vi "GE5565 Enable DMA Interrupt (Cluster) Multi.vi"(4 "error in (no error)":errorcluster, 6 "transfer size (1024 bytes)":u32=1024, 7 "VMIC reference in":T1) -> (0 "error out":errorcluster, 3 "VMIC reference out":T1)   [LabVIEW 2020, in "RefMem DMA Engine.lvlib"]
uses:
  RefMem DMA Engine.lvlib
  <vilib>/Instr/_visa.llb/Select Event Type.ctl
  <vilib>/Instr/_visa.llb/VISA Register Access Address Space.ctl
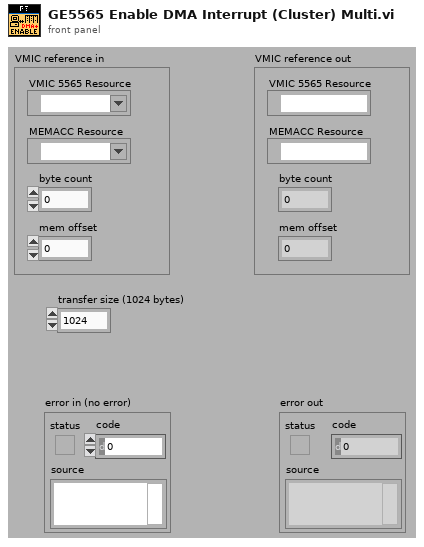
[diagram p1: front panel]
types:
  T1 = cluster{"VMIC 5565 Resource":refnum<visa-resource-name>, "MEMACC Resource":refnum<visa-resource-name>, "byte count":u32, "mem offset":u32}
  T2 = typedef "Select Event Type.ctl" = u32
  T3 = typedef "VISA Register Access Address Space.ctl" = u16
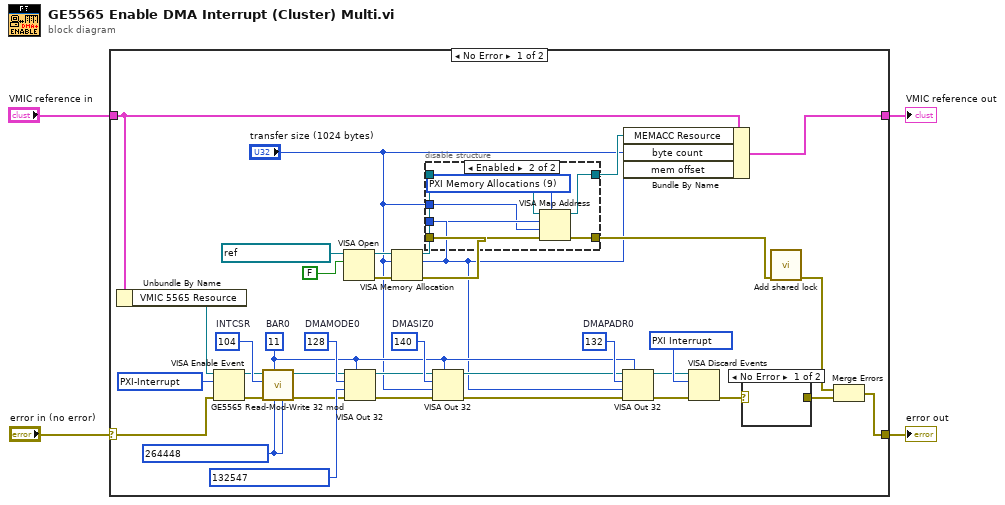
[diagram p0: block diagram]
diagram:
  n1 = case shown="No Error" "error in (no error)" {
    selector: "error in (no error)" -> [w27 w52]
    tunnel: "VMIC reference in" -> [w18 w53]
    tunnel: [w17 w53] -> w1
    tunnel: [w29 w52] -> w3
    frame No Error {
      w25 = u16 11  # BAR0
      w16 = T2 1073684514 items=["Service Request"=1073684491, "Trigger"=3221168138, "Clear"=1073684493, "VXI Signal"=1073684512, "VXI/VME Interrupt"=3221168161, "VXI/VME Sysfail"=1073684509, "VXI/VME Sysreset"=1073684510, "GPIB CIC"=1073684498, "GPIB Talk"=1073684499, "GPIB Listen"=1073684500, "PXI Interrupt"=1073684514, "Serial Break"=1073684515, "Serial TermChar"=1073684516, "Serial CTS"=1073684521, "Serial DSR"=1073684522, "Serial DCD"=1073684524, "Serial RI"=1073684526, "Serial Character"=1073684533, "USB Interrupt"=1073684535, "All Enabled"=1073709055] ("Event Type")
      w26 = u32 104  # INTCSR
      w24 = u32 264448 ("value")
      w28 = T2 1073684514 items=["ServiceRequest"=1073684491, "Trigger"=3221168138, "Clear"=1073684493, "VXI-Signal"=1073684512, "VXI/VME-Interrupt"=3221168161, "VXI/VME-Sysfail"=1073684509, "VXI/VME-Sysreset"=1073684510, "GPIB-CIC"=1073684498, "GPIB-Talk"=1073684499, "GPIB-Listen"=1073684500, "PXI-Interrupt"=1073684514, "AllEnabled"=1073709055] ("Event Type")
      w32 = u32 132  # DMAPADR0
      w35 = u32 140  # DMASIZ0
      w37 = u32 128  # DMAMODE0
      n2 = Unbundle By Name(w18) -> ("VMIC 5565 Resource"=w19:refnum<visa-resource-name>)
      n3 = VISA Enable Event(8:w27, 10:w28, 11:w19) -> (0:w23:errorcluster, 3:w22:refnum<visa-resource-name>)  [unwired: 1 in]
      n4 = call "GE5565 Read-Mod-Write 32 mod.vi"("value"=w24, "inv bit mask"=w24, "address space (13: BAR2)"=w25, "error in (no error)"=w23, "offset (0)"=w26, "VISA resource name"=w22) -> ("error out"=w20:errorcluster, "VISA resource name out"=w21:refnum<visa-resource-name>)  [unwired: 4 in]
      n5 = VISA Open(duplicate session (F)=FALSE, VISA resource name=refnum<visa-resource-name> "PXI0::MEMACC") -> (VISA resource name=w40:refnum<visa-resource-name>, error out=w41:errorcluster)  [unwired: 3 in]
      n6 = VISA Out 32(7:w25, 8:w20, 9:u32 132547 ("value (0)"), 10:w37, 11:w21) -> (0:w34:errorcluster, 3:w33:refnum<visa-resource-name>)
      n7 = VISA Memory Allocation(8:w41, 10:"transfer size (1024 bytes)", 11:w40) -> (0:w8:errorcluster, 2:w6:u32, 3:w9:refnum<visa-resource-name>)
      n8 = disable-structure shown="Enabled" {
        disable-tunnel: [w43 w47] -> w10
        disable-tunnel: w9 -> [w43 w48]
        disable-tunnel: w8 -> [w42 w49]
        disable-tunnel: [w42 w50] -> w7
        disable-tunnel: w6 -> [_ w46]
        disable-tunnel: "transfer size (1024 bytes)" -> [_ w45]
        frame Disabled {
        }
        frame Enabled {
          w44 = T3 9 items=["VXI/VME A16"=1, "VXI/VME A24"=2, "VXI/VME A32"=3, "VXI/VME A64"=4, "PXI Memory Allocations"=9, "PXI Configuration"=10, "PXI BAR0"=11, "PXI BAR1"=12, "PXI BAR2"=13, "PXI BAR3"=14, "PXI BAR4"=15, "PXI BAR5"=16] ("Address Space")
          n9 = VISA Map Address(7:w44, 8:w49, 9:w45, 10:w46, 11:w48) -> (0:w50:errorcluster, 3:w47:refnum<visa-resource-name>)  [unwired: 1 in]
        }
      }
      n10 = VISA Out 32(7:w25, 8:w34, 9:"transfer size (1024 bytes)", 10:w35, 11:w33) -> (0:w30:errorcluster, 3:w31:refnum<visa-resource-name>)
      n11 = VISA Out 32(7:w25, 8:w30, 9:w6, 10:w32, 11:w31) -> (0:w14:errorcluster, 3:w15:refnum<visa-resource-name>)
      n12 = Bundle By Name(cluster=w18, "MEMACC Resource"=w10, "byte count"="transfer size (1024 bytes)", "mem offset"=w6) -> (w17:T1)
      n13 = VISA Discard Events(8:w14, 10:w16, 11:w15) -> (0:w13:errorcluster)  [unwired: 1 in, 1 out]
      n14 = case shown="No Error" w13 {
        selector: w13 -> [_ w51]
        tunnel: [_ w51] -> w12
        frame No Error {
        }
        frame Error {
        }
      }
      n15 = call "Add shared lock.vi"("error in (no error)"=w7) -> ("error out"=w11:errorcluster)  [unwired: 10 in]
      n16 = Merge Errors(w11, w12) -> (w29:errorcluster)
    }
    frame Error {
    }
  }
  "error out" <- w3
  "VMIC reference out" <- w1
